vi "Work.vi"(8 "error in (no error)":errorcluster, 9 "Outputs":refnum<class "Output.lvclass">[](array[class]), 10 "Inputs":refnum<class "Input.lvclass">[](array[class]), 11 "WaveSourceBlock in":refnum<class "WaveSourceBlock.lvclass">) -> (0 "error out":errorcluster, 3 "WaveSourceBlock out":refnum<class "WaveSourceBlock.lvclass">)   [LabVIEW 2020, in "WaveSourceBlock.lvclass"]
uses:
  WaveSourceBlock.lvclass
  Parallel Block/Input/Input.lvclass
  Parallel Block/Output/Output.lvclass
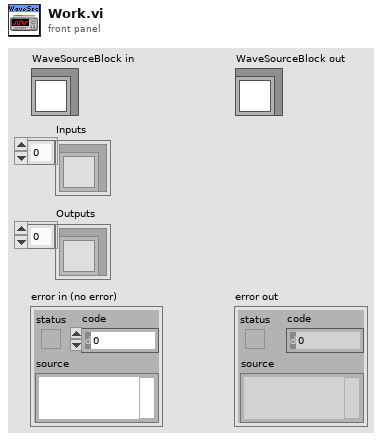
[diagram p1: front panel]
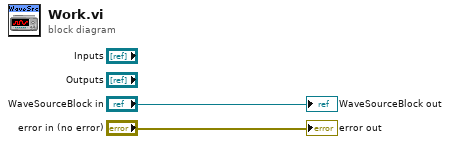
[diagram p0: block diagram]
diagram:
  "error out" <- "error in (no error)"
  "WaveSourceBlock out" <- "WaveSourceBlock in"
